vi "PrepareNotification.vi"(8 "error in (no error)":errorcluster, 11 "WeatherData in":refnum<class "Weather Station.lvclass">) -> (0 "error out":errorcluster, 3 "WeatherData out":refnum<class "Weather Station.lvclass">)   [LabVIEW 2020, in "Weather Station.lvclass"]
uses:
  Weather Station.lvclass
  C:/Users/fflores/Documents/GitHub Projects/OOP-Concepts-in-LabVIEW/Relations Between Objects/Inheritance/Observer Pattern Example/Observable/Observable.lvclass
  Weather Station.lvclass/Weather Station.ctl
  Observer/Observer.lvclass/Observer.ctl
  Observable/Observable.lvclass/Observable.ctl
  Observer/Observer.lvclass
  Observable/Observable.lvclass
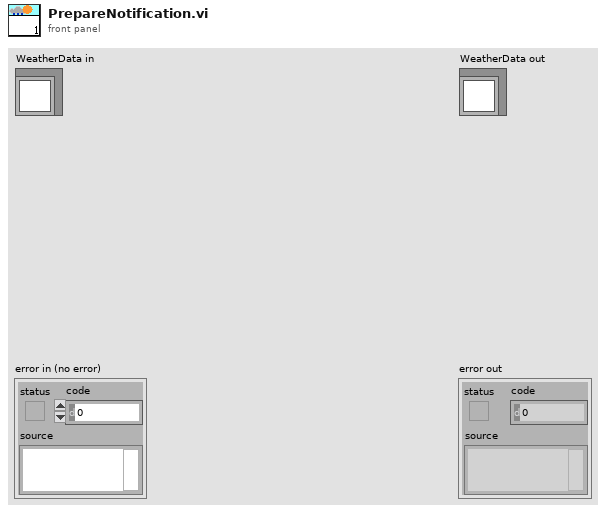
[diagram p1: front panel]
types:
  T1 = cluster{"Temperature":dbl, "Humidity":dbl, "Pressure":dbl, "Stop?":bool}
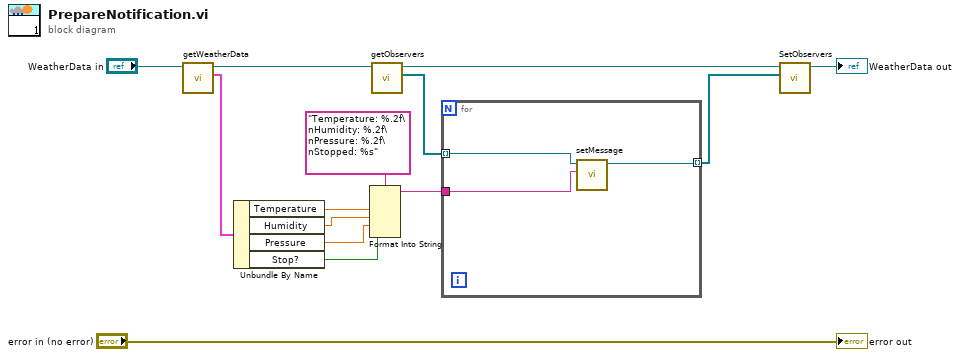
[diagram p0: block diagram]
diagram:
  n1 = call "getWeatherData.vi"("WeatherData in"="WeatherData in") -> ("WeatherData"=w7:T1, "WeatherData out"=w12:refnum<class "Weather Station.lvclass">)  [unwired: 8 in, 1 out]
  n2 = Unbundle By Name(w7) -> ("Temperature"=w5:dbl, "Humidity"=w4:dbl, "Pressure"=w3:dbl, "Stop?"=w2:bool)
  n3 = Format Into String(format string="Temperature: %.2f\nHumidity: %.2f\nPressure: %.2f\nStopped: %s", w5, w4, w3, w2) -> (resulting string=w1:string)  [unwired: 2 in, 1 out]
  n4 = call-dynamic "getObservers.vi"("Observable in"=w12) -> ("Observers"=w10:refnum<class "Observer.lvclass">[], "Observable out"=w11:refnum<class "Weather Station.lvclass">)  [unwired: 8 in, 1 out]
  n5 = for {
    tunnel: w10 -> [w17] mode=indexing
    tunnel: [w16] -> w8 mode=indexing
    tunnel: w1 -> [w15]
    n6 = call "setMessage.vi"("Message"=w15, "Observer in"=w17) -> ("Observer out"=w16:refnum<class "Observer.lvclass">)  [unwired: 8 in, 1 out]
  }
  n7 = call "SetObservers.vi"("Observers"=w8, "Observable in"=w11) -> ("Observable out"=→"WeatherData out":refnum<class "Weather Station.lvclass">)  [unwired: 8 in, 1 out]
  "error out" <- "error in (no error)"
